vi "Degrees To Correct Target.vi"(8 "error in":errorcluster, 10 "Distance to Wall (ft)":dbl) -> (0 "error out":errorcluster, 2 "Degrees":dbl)   [LabVIEW 2013]
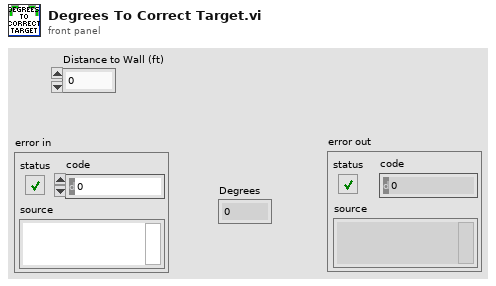
[diagram p1: front panel]
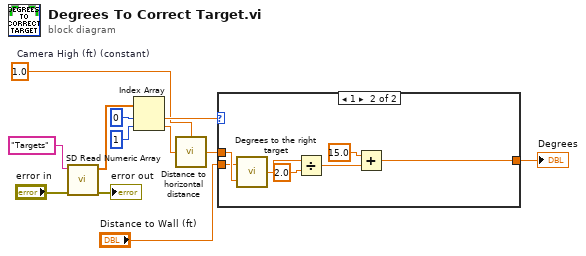
[diagram p0: block diagram]
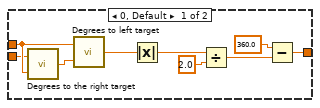
[diagram p2: hidden frame]
diagram:
  w3 = 1.0  # Camera High (ft) (constant)
  n1 = call <vilib>:"SD Read Numeric Array.vi"("error in"="error in", "Name"="Targets") -> ("error out"=→"error out":errorcluster, "Numeric Array"=w2:dbl[])  [unwired: 7 in, 1 out]
  n2 = Index Array(array=w2, index #1=0 ("index"), index #2=1 ("index")) -> (element #1=w9:dbl, element #2=w5:dbl)
  n3 = call "Distance to horizontal distance.vi"("Camera High (ft) (constant)"=w3, "Distance (ft)"=w5) -> ("Horizontal Distance (ft)"=w8:dbl)  [unwired: 2 in]
  n4 = case shown="1" w9 {
    tunnel: w8 -> [w20 w28]
    tunnel: [w15 w22] -> w1
    tunnel: "Distance to Wall (ft)" -> [w19 w27]
    frame 0, Default {
      n5 = call "Degrees to the right target.vi"("Distance to Target (ft)"=w20, "Distance to Wall (ft)"=w19) -> ("Degrees to Right Target"=w21:dbl)
      n6 = call "Degrees to left target.vi"("Degrees From The Right Target"=w21, "d"=w20) -> ("Degrees To The Left Target"=w16:dbl)
      n7 = Absolute Value(x=w16) -> (abs(x)=w13:dbl)
      n8 = Divide(x=w13, y=2.0) -> (x/y=w14:dbl)
      n9 = Subtract(x=360.0, y=w14) -> (x-y=w15:dbl)
    }
    frame 1 {
      n10 = call "Degrees to the right target.vi"("Distance to Target (ft)"=w28, "Distance to Wall (ft)"=w27) -> ("Degrees to Right Target"=w25:dbl)
      n11 = Divide(x=w25, y=2.0) -> (x/y=w24:dbl)
      n12 = Add(x=15.0, y=w24) -> (x+y=w22:dbl)
    }
  }
  "Degrees" <- w1
